vi "tt.vi"() -> ()   [LabVIEW 2013]
uses:
  <vilib>/Instr/_visa.llb/VISA Configure Serial Port (Instr).vi
panel:
  in  "termination char\n(0xA = '\\n' = LF)":u8=10 format="%.0x"
  in  "Angle":string
  in  "stop":bool
  in  "Send":bool
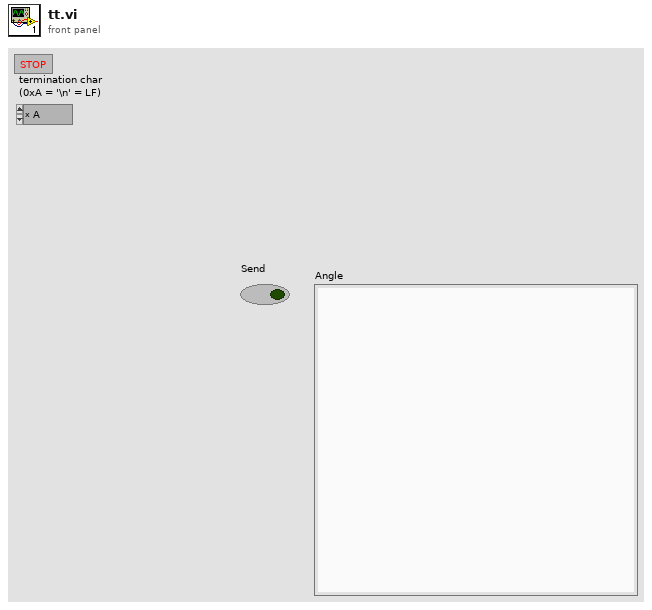
[diagram p1: front panel]
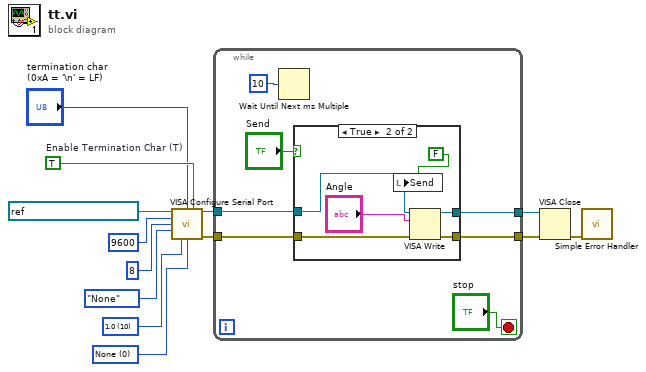
[diagram p0: block diagram]
diagram:
  w2 = TRUE  # Enable Termination Char (T)
  w12 = u16 10 items=["1.0"=10, "1.5"=15, "2.0"=20] ("stop bits (10: 1 bit)")
  w11 = u16 0 items=["None", "XON/XOFF", "RTS/CTS", "XON/XOFF & RTS/CTS", "DTR/DSR", "XON/XOFF & DTR/DSR"] ("flow control (0:none)")
  n1 = call-poly "VISA Configure Serial Port"("VISA resource name"=refnum<visa-resource-name> "COM14", "termination char\n(0xA = '\\n' = LF)"="termination char\n(0xA = '\\n' = LF)", "Enable Termination\nChar (T)"=w2, "baud rate (9600)"=u32 9600, "data bits (8)"=u16 8, "parity (0:none)"=enum16{"None", "Odd", "Even", "Mark", "Space"}."None", "stop bits (10: 1 bit)"=w12, "flow control (0:none)"=w11) -> ("VISA resource name out"=w6:refnum<visa-resource-name>, "error out"=w7:errorcluster)  [unwired: 6 in]
  n2 = while {
    tunnel: w7 -> [w17]
    tunnel: w6 -> [w16]
    tunnel: [w15] -> w4
    tunnel: [w14] -> w3
    stop <- "stop" stop-if-true
    n3 = Wait Until Next ms Multiple(millisecond multiple=u32 10 ("milliseconds to wait")) -> ()  [unwired: 1 out]
    n4 = case shown="True" "Send" {
      tunnel: w17 -> [w22 w27]
      tunnel: w16 -> [w21 w26]
      tunnel: [w21 w25] -> w15
      tunnel: [w22 w24] -> w14
      frame False {
      }
      frame True {
        n5 = local write "Send"(FALSE ("Send")) -> ()
        n6 = VISA Write(VISA resource name=w26, write buffer="Angle", error in (no error)=w27) -> (VISA resource name out=w25:refnum<visa-resource-name>, error out=w24:errorcluster)  [unwired: 1 out]
      }
    }
  }
  n7 = VISA Close(VISA resource name=w4, error in (no error)=w3) -> (error out=w5:errorcluster)
  n8 = call <vilib>:"Simple Error Handler.vi"("error in (no error)"=w5) -> ()  [unwired: 4 in, 5 out]
